vi "AttackPsSkill.vi"(9 "Game in":refnum<class "Game.lvclass">, 10 "Robot":refnum<class "Robot.lvclass">, 11 "AttackPsSkill in":refnum<class "AttackPsSkill.lvclass">) -> (2 "Robot out":refnum<class "Robot.lvclass">, 3 "AttackPsSkill out":refnum<class "AttackPsSkill.lvclass">)   [LabVIEW 2020, in "AttackPsSkill.lvclass"]
uses:
  AttackPsSkill.lvclass
  Robot_class/Robot.lvclass
  Game_class/Game.lvclass
  Game_class/Game.lvclass/Game.ctl
  Object_class/Object.lvclass/Object.ctl
  Robot_class/Robot.lvclass/Robot.ctl
  <vilib>/Analysis/_algsub.llb/Real Vector Norm.vi
  Game_class/Read BallRef.vi
  Game_class/Read FieldRef.vi
  Object_class/Read y.vi
  Object_class/Read x.vi
  Robot_class/Write dest_x.vi
  Robot_class/Write dest_y.vi
  Robot_class/Write dest_orientation.vi
  Robot_class/Write kick_x.vi
  Ball_class/Ball.lvclass
  C:/Users/Pedro/Dropbox/My PC (LAPTOP-06JBDO7V)/Documents/GitHub/SSL_AI/Object_class/Object.lvclass
  Field_class/Field.lvclass
  <vilib>/Analysis/NI_AALPro.lvlib
panel:
  out "error out 2":errorcluster
  in  "error in (no error) 2":errorcluster
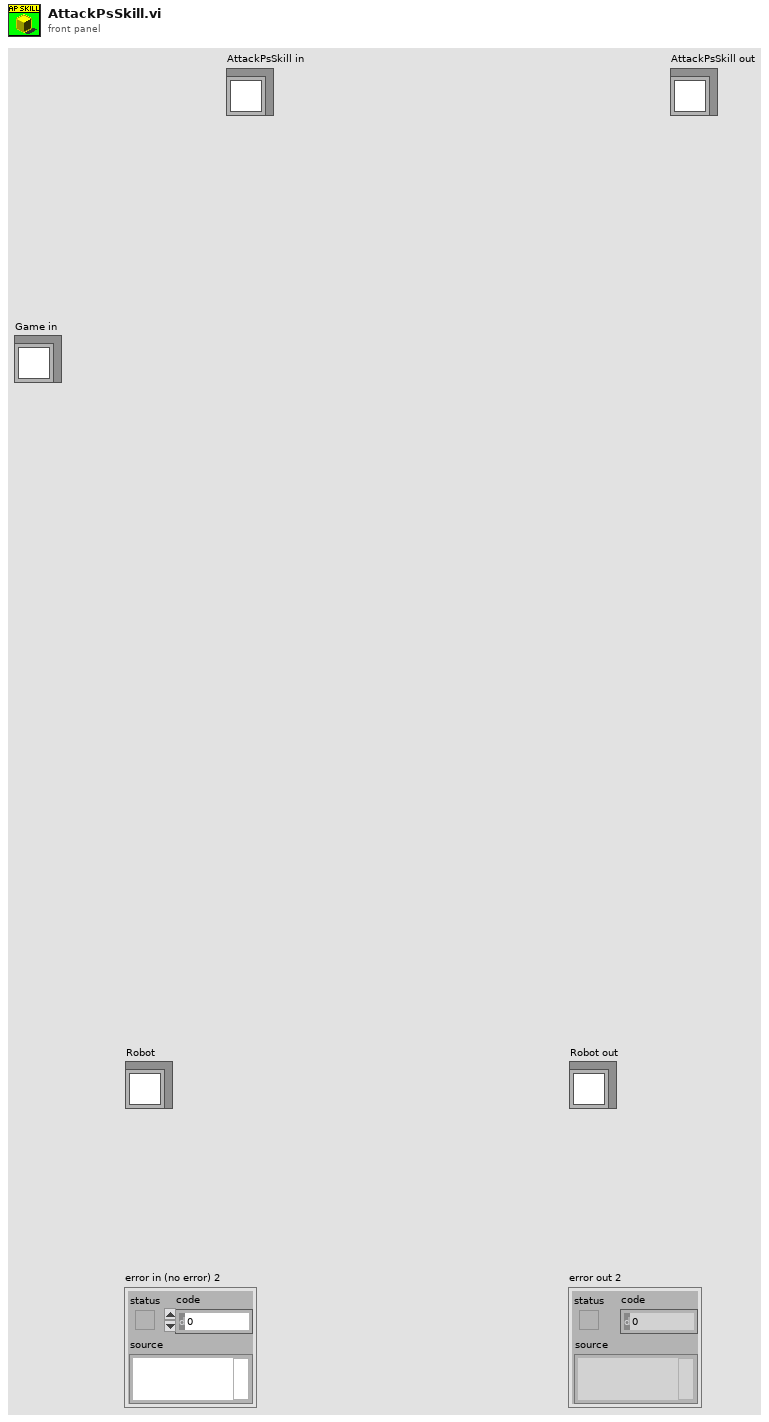
[diagram p1: front panel]
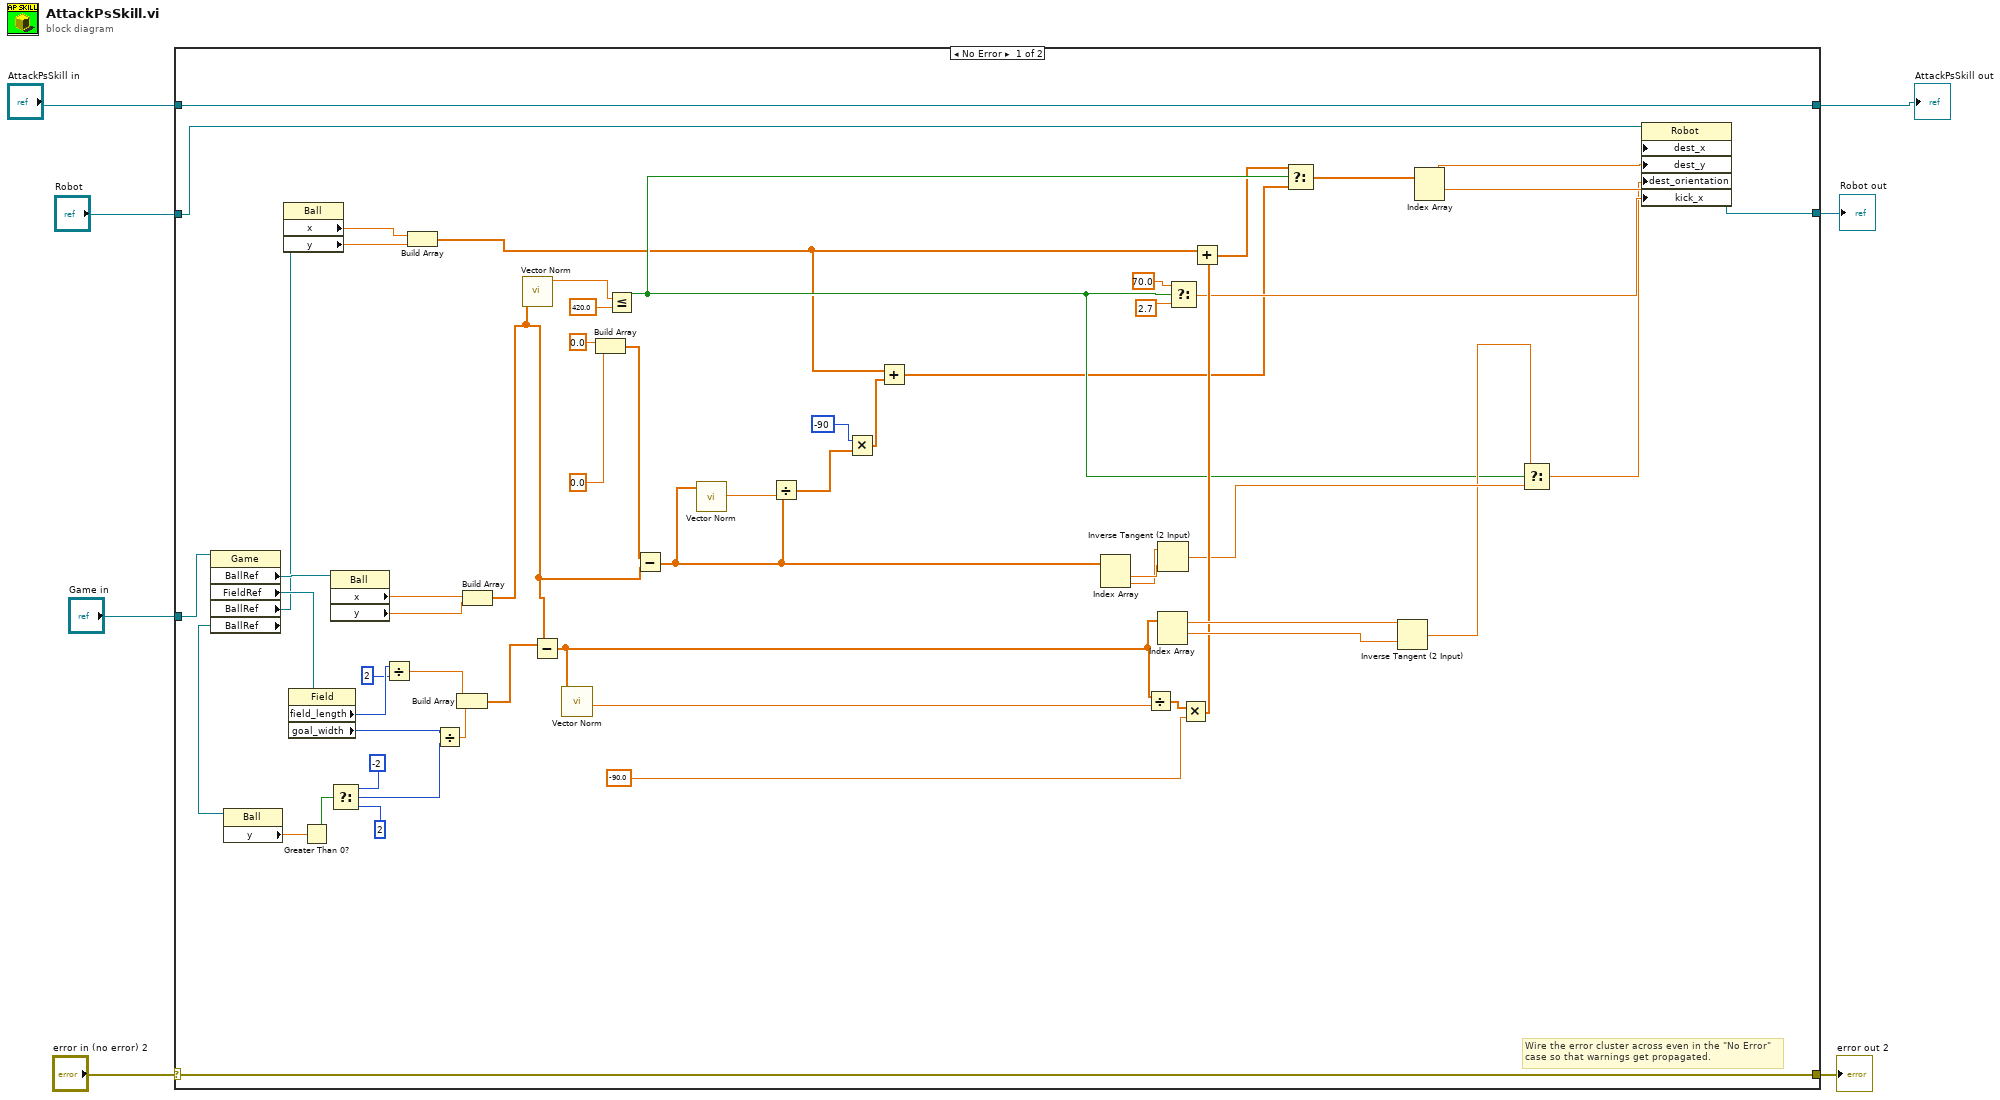
[diagram p0: block diagram]
diagram:
  n1 = case shown="No Error" "error in (no error) 2" {
    selector: "error in (no error) 2" -> [w63 w67]
    tunnel: [w63 w67] -> w6
    tunnel: [w64 w66] -> w3
    tunnel: "AttackPsSkill in" -> [w64 w66]
    tunnel: "Robot" -> [w62 w65]
    tunnel: [w61 w65] -> w4
    tunnel: "Game in" -> [w60 _]
    frame No Error {
      # "Wire the error cluster across even in the \"No Error\"\ncase so that warnings get propagated."
      n2 = property class="Game"(reference=w60) -> ("BallRef"=w59:refnum<class "Ball.lvclass">, "FieldRef"=w58:refnum<class "Field.lvclass">, "BallRef"=w49:refnum<class "Ball.lvclass">, "BallRef"=w48:refnum<class "Ball.lvclass">)  [unwired: 1 in, 2 out]
      n3 = property class="Ball"(reference=w48) -> ("y"=w47:dbl)  [unwired: 1 in, 2 out]
      n4 = property class="Ball"(reference=w49) -> ("x"=w39:dbl, "y"=w38:dbl)  [unwired: 1 in, 2 out]
      n5 = property class="Field"(reference=w58) -> ("field_length"=w57:i32, "goal_width"=w42:i32)  [unwired: 1 in, 2 out]
      n6 = Greater Than 0?(x=w47) -> (x > 0?=w46:bool)
      n7 = property class="Ball"(reference=w59) -> ("x"=w54:dbl, "y"=w53:dbl)  [unwired: 1 in, 2 out]
      n8 = Select(t=-2 ("x"), s=w46, f=2 ("x")) -> (s? t:f=w43:i32)
      n9 = Divide(x=w57, y=2) -> (x/y=w56:dbl)
      n10 = Build Array(w39, w38) -> (w11:dbl[])
      n11 = Divide(x=w42, y=w43) -> (x/y=w55:dbl)
      n12 = Build Array(w56, w55) -> (w32:dbl[])
      n13 = Build Array(w54, w53) -> (w18:dbl[])
      n14 = call-poly <vilib>:"Vector Norm.vi"("Input Vector"=w18) -> ("norm"=w28:dbl)  [unwired: 9 in, 1 out]
      n15 = Subtract(x=w32, y=w18) -> (x-y=w34:dbl[])
      n16 = call-poly <vilib>:"Vector Norm.vi"("Input Vector"=w34) -> ("norm"=w33:dbl)  [unwired: 9 in, 1 out]
      n17 = Build Array(0.0 ("element"), 0.0 ("element")) -> (w19:dbl[])
      n18 = Less Or Equal?(x=w28, y=420.0) -> (x <= y?=w17:bool)
      n19 = Subtract(x=w19, y=w18) -> (x-y=w16:dbl[])
      n20 = call-poly <vilib>:"Vector Norm.vi"("Input Vector"=w16) -> ("norm"=w15:dbl)  [unwired: 9 in, 1 out]
      n21 = Divide(x=w16, y=w15) -> (x/y=w14:dbl[])
      n22 = Multiply(x=-90, y=w14) -> (x*y=w12:dbl[])
      n23 = Add(x=w11, y=w12) -> (x+y=w10:dbl[])
      n24 = Index Array(array=w16) -> (element #1=w26:dbl, element #2=w25:dbl)  [unwired: 2 in]
      n25 = Divide(x=w34, y=w33) -> (x/y=w41:dbl[])
      n26 = Index Array(array=w34) -> (element #1=w51:dbl, element #2=w50:dbl)  [unwired: 2 in]
      n27 = Inverse Tangent (2 Input)(1:w26, 2:w25) -> (0:w24:dbl)
      n28 = Select(t=70.0, s=w17, f=2.7) -> (s? t:f=w29:dbl)
      n29 = Multiply(x=w41, y=-90.0) -> (x*y=w37:dbl[])
      n30 = Add(x=w11, y=w37) -> (x+y=w9:dbl[])
      n31 = Select(t=w9, s=w17, f=w10) -> (s? t:f=w8:dbl[])
      n32 = Inverse Tangent (2 Input)(1:w51, 2:w50) -> (0:w23:dbl)
      n33 = Index Array(array=w8) -> (element #1=w36:dbl, element #2=w35:dbl)  [unwired: 2 in]
      n34 = Select(t=w23, s=w17, f=w24) -> (s? t:f=w22:dbl)
      n35 = property class="Robot"(reference=w62, "dest_x"=w36, "dest_y"=w35, "dest_orientation"=w22, "kick_x"=w29) -> (reference out=w61:refnum<class "Robot.lvclass">)  [unwired: 1 in, 1 out]
    }
    frame Error {
    }
  }
  "AttackPsSkill out" <- w3
  "error out 2" <- w6
  "Robot out" <- w4
